vi "VI Tree.vi"   [LabVIEW 2016]
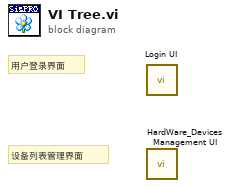
[diagram p0: block diagram]
diagram:
  # "设备列表管理界面"
  # "用户登录界面"
  n1 = call "Login UI.vi"() -> ()  [unwired: 12 in]
  n2 = call "HardWare_Devices Management UI.vi"() -> ()  [unwired: 12 in]
